vi "Set Method End Time.vi"(9 "Method Start Time":timestamp, 10 "Test Method Name":string, 11 "Test Case Result In":T1) -> (3 "Test Case Result Out":T1)   [LabVIEW 2020, in "Test Case Result.lvlib"]
uses:
  Test Case Result.lvlib
  Assertion Result/Public/TypeDefs/Status.ctl
  Assertion Result/Assertion Result.lvlib
  Assertion Result/Public/TypeDefs/Assertion Type.ctl
  Assertion Result/Assertion Result.ctl
  Method Result/Method Result.ctl
  Method Result/Method Result.lvlib
  Test Case Result.ctl
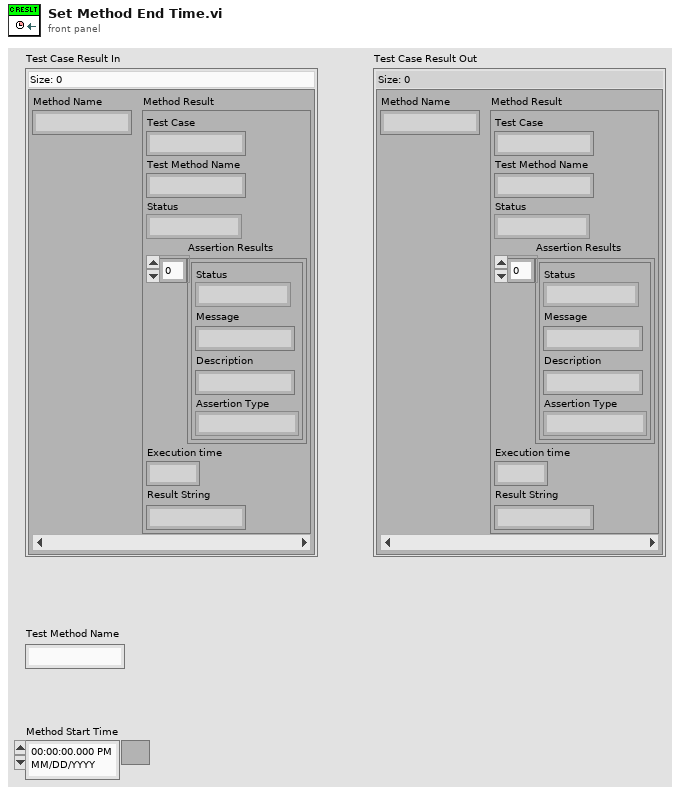
[diagram p1: front panel]
types:
  T1 = typedef "Test Case Result.lvlib/Test Case Result.ctl" = map{string, T2}
  T2 = typedef "Method Result.lvlib/Method Result.ctl" = cluster{"Test Case":string, "Test Method Name":string, "Status":T3, "Assertion Results":T4[], "Execution time":dbl, "Result String":string}
  T3 = typedef "Assertion Result.lvlib/Status.ctl" = enum16{"Pass", "Fail", "Error", "Skipped", "Setup Error", "Broken", "Teardown Error"}
  T4 = typedef "Assertion Result.lvlib/Assertion Result.ctl" = cluster{"Status":T3, "Message":string, "Description":string, "Assertion Type":T5}
  T5 = typedef "Assertion Result.lvlib/Assertion Type.ctl" = enum16{"None", "Pass", "Fail", "Skip", "Pass if Equal", "Fail if Equal", "Pass if Error", "Fail if Error", "Pass if", "Fail if"}
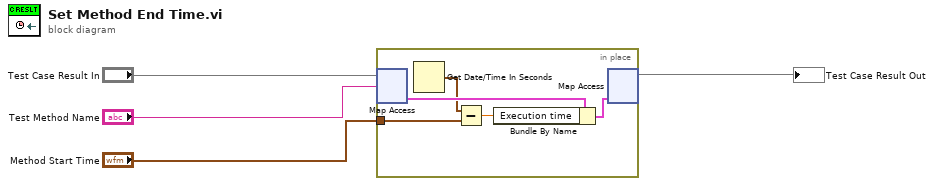
[diagram p0: block diagram]
diagram:
  n1 = in-place {
    in-place-border: "Method Start Time" -> [w9]
    n2 = in-place-map #1("Test Case Result In", "Test Method Name") -> (w8:T2)  [unwired: 1 in, 1 out]
    n3 = Get Date/Time In Seconds() -> (seconds since 1Jan1904=w5:timestamp)
    n4 = Subtract(x=w5, y=w9) -> (x-y=w6:dbl)
    n5 = Bundle By Name(cluster=w8, "Execution time"=w6) -> (w7:T2)
    n6 = in-place-map #1(w7) -> (→"Test Case Result Out":T1)  [unwired: 1 in, 2 out]
  }
